vi "Do.vi"(8 "error in (no error)":errorcluster, 10 "Actor in":refnum<class "Actor.lvclass">, 11 "Open File Msg":refnum<class "Open File Msg.lvclass">) -> (0 "error out":errorcluster, 2 "Actor out":refnum<class "Actor.lvclass">)   [LabVIEW 2020, in "File Writer.lvlib" / "Open File Msg.lvclass"]
doc: "This Do implementation will execute Core and then Respond on Data and lastly Publish Data if this is not handled on the sender."
uses:
  Open File Msg.lvclass
  C:/Current projects/WS/PPL/HDH.Actor Framework.Core.Publisher.lvlibp/Messages/Response Msg/Response Msg.lvclass
  PPL/HDH.Actor Framework.Core.Actor.lvlibp/1abvi3w/vi.lib/ActorFramework/Actor/Actor.lvclass
  File Writer/File Writer.lvclass
  Open File Msg.lvclass/Open File Msg.ctl
  PPL/HDH.Actor Framework.Core.Publisher.lvlibp/Messages/Response Msg/Response Msg.lvclass
  File Writer.lvlib
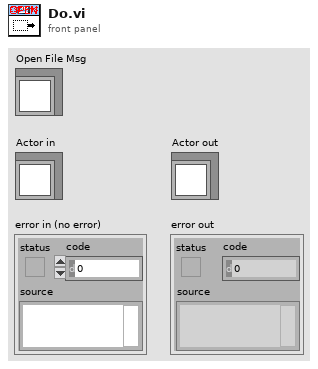
[diagram p1: front panel]
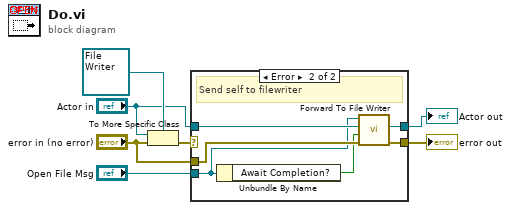
[diagram p0: block diagram]
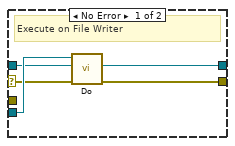
[diagram p2: hidden frame]
diagram:
  n1 = To More Specific Class(target class=refnum<class "File Writer.lvclass"> refnum ("File Writer.lvlib:File Writer.lvclass"), reference="Actor in", error in="error in (no error)") -> (error out=w7:errorcluster)  [unwired: 1 out]
  n2 = case shown="Error" w7 {
    selector: w7 -> [w8 _]
    tunnel: [w12 w16] -> w2
    tunnel: [w11 w15] -> w1
    tunnel: "Open File Msg" -> [w10 w14]
    tunnel: "Actor in" -> [w9 w17]
    tunnel: "error in (no error)" -> [_ w18]
    frame No Error {
      # "Execute on File Writer"
      n3 = call-parent "Do.vi"("error in (no error)"=w8, "Actor in"=w9, "Response Msg"=w10) -> ("error out"=w12:errorcluster, "Actor out"=w11:refnum<class "Actor.lvclass">)  [unwired: 7 in]
    }
    frame Error {
      # "Send self to filewriter"
      n4 = Unbundle By Name(w14) -> ("Await Completion?"=w13:bool)
      n5 = call "Forward To File Writer.vi"("error in (no error)"=w18, "Await Completion?"=w13, "Actor in"=w17, "Response Msg in"=w14) -> ("error out"=w16:errorcluster, "Actor out"=w15:refnum<class "Actor.lvclass">)  [unwired: 6 in]
    }
  }
  "error out" <- w2
  "Actor out" <- w1
